vi "cXB_trt-3-sta.vi"(2 "errout":errorcluster caption="err in", 3 "cX":T1) -> (0 "err out":errorcluster, 1 "cX-s":T1)   [LabVIEW 2010]
uses:
  lv_04/commandes/cX.ctl
  lv_04/commandes/cSTA_varid.ctl
  lv_04/commandes/c_TDMS_ch_variable.ctl
  lv_04/commandes/c_TDMS_ch_donnees.ctl
  lv_04/commandes/c0-var-n.ctl
  lv_04/commandes/cSTA_num_do_cr.ctl
  lv_04/commandes/c02-do-num.ctl
  lv_04/commandes/c04-stat-num.ctl
  lv_04/commandes/cSTA_txt_do_cr.ctl
  lv_04/commandes/c02-do-txt.ctl
  lv_04/commandes/c04-stat-txt.ctl
  lv_04/commandes/cSTA_dist.ctl
  lv_04/commandes/c03-dist-S.ctl
  lv_04/commandes/c0-dist-xy.ctl
  lv_04/commandes/c03-dist-T.ctl
  lv_04/commandes/c03-dist-SPC.ctl
  lv_04/lv_04.lvlib
  lv_01/lv_01.lvlib
  lv_02/lv_02.lvlib
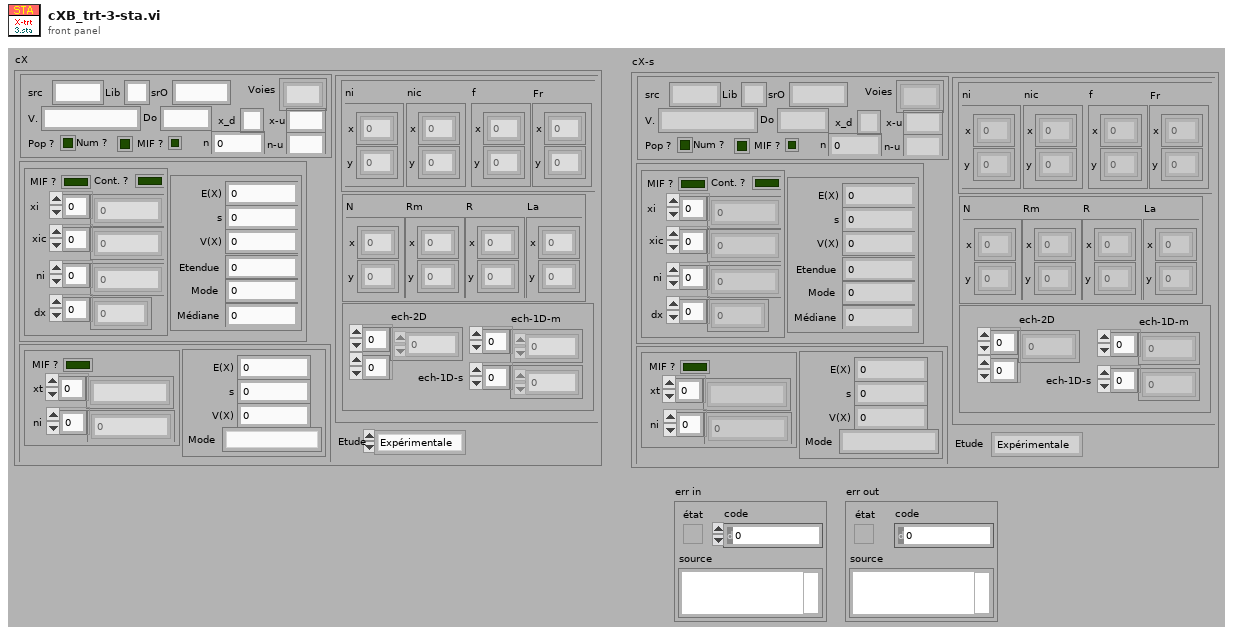
[diagram p1: front panel]
types:
  T1 = typedef "lv_04.lvlib/cX.ctl" = cluster{"src":T2, "num":T6, "txt":T9, "dist":T12, "Etude":enum16{"Expérimentale", "Modèle"}}
  T2 = typedef "lv_04.lvlib/cSTA_varid.ctl" = cluster{"src":string, "Lib":string, "srO":string, "V.":T3, "Voies":string[], "Do":T4, "n":T5, "Num ?":bool, "Pop ?":bool, "x_d":string, "x-u":string, "n-u":string, "MIF ?":bool}
  T3 = typedef "lv_04.lvlib/c_TDMS_ch_variable.ctl" = string
  T4 = typedef "lv_04.lvlib/c_TDMS_ch_donnees.ctl" = string
  T5 = typedef "lv_04.lvlib/c0-var-n.ctl" = i32
  T6 = typedef "lv_04.lvlib/cSTA_num_do_cr.ctl" = cluster{"do":T7, "sta":T8}
  T7 = typedef "lv_04.lvlib/c02-do-num.ctl" = cluster{"MIF ?":bool, "Cont. ?":bool, "xi":dbl[], "xic":dbl[], "ni":u32[], "dx":dbl[]}
  T8 = typedef "lv_04.lvlib/c04-stat-num.ctl" = cluster{"E(X)":dbl, "s":dbl, "V(X) ":dbl, "Etendue":dbl, "Mode":dbl, "Médiane":dbl}
  T9 = typedef "lv_04.lvlib/cSTA_txt_do_cr.ctl" = cluster{"do":T10, "sta":T11}
  T10 = typedef "lv_04.lvlib/c02-do-txt.ctl" = cluster{"xt":string[], "ni":dbl[], "MIF ?":bool}
  T11 = typedef "lv_04.lvlib/c04-stat-txt.ctl" = cluster{"E(X)":dbl, "s":dbl, "V(X) ":dbl, "Mode":string}
  T12 = typedef "lv_04.lvlib/cSTA_dist.ctl" = cluster{"S":T13, "T":T15, "spc":T16}
  T13 = typedef "lv_04.lvlib/c03-dist-S.ctl" = cluster{"nic":T14, "f":T14, "Fr":T14, "ni":T14}
  T14 = typedef "lv_04.lvlib/c0-dist-xy.ctl" = cluster{"x":dbl[], "y":dbl[]}
  T15 = typedef "lv_04.lvlib/c03-dist-T.ctl" = cluster{"N":T14, "Rm":T14, "R":T14, "La":T14}
  T16 = typedef "lv_04.lvlib/c03-dist-SPC.ctl" = cluster{"ech-2D":dbl[][], "ech-1D-m":dbl[], "ech-1D-s":dbl[]}
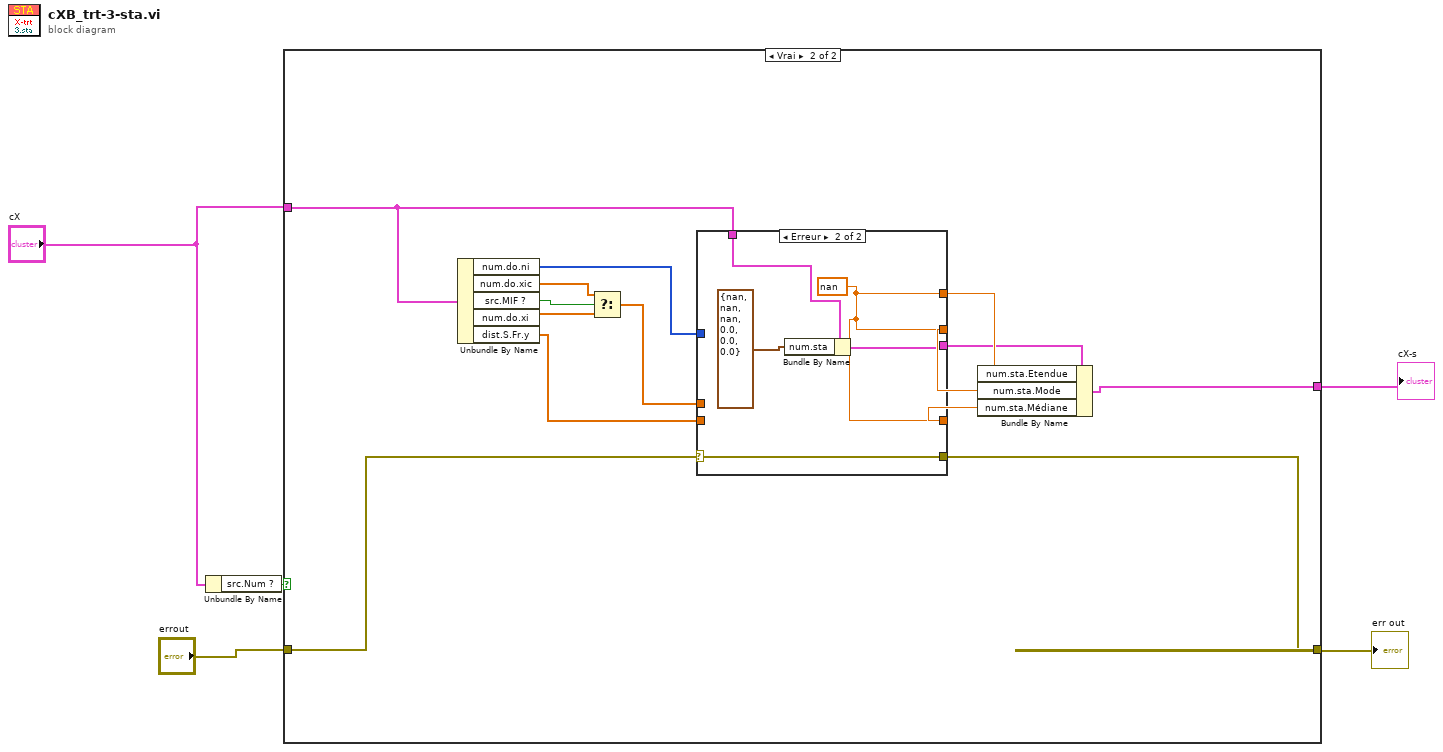
[diagram p0: block diagram]
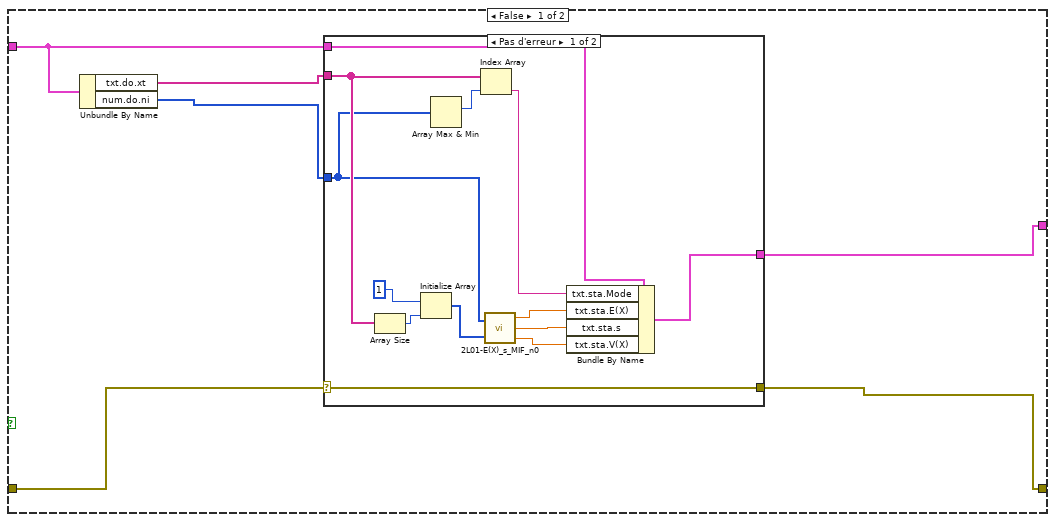
[diagram p2: hidden frame]
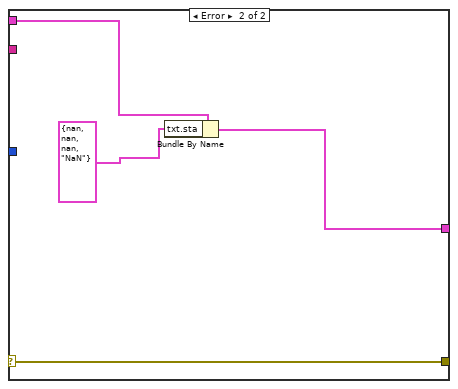
[diagram p3: hidden frame]
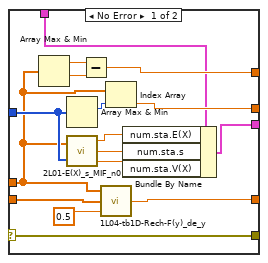
[diagram p4: hidden frame]
diagram:
  n1 = Unbundle By Name("cX") -> ("src.Num ?"=w3:bool)
  n2 = case shown="Vrai" w3 {
    tunnel: "errout" -> [w8 w30]
    tunnel: [w7 w29] -> w4
    tunnel: "cX" -> [w9 w32]
    tunnel: [w6 w33] -> w1
    frame False {
      n3 = Unbundle By Name(w9) -> ("txt.do.xt"=w11:string[], "num.do.ni"=w10:u32[])
      n4 = case shown="Pas d'erreur" w8 {
        selector: w8 -> [w23 w28]
        tunnel: [w12 w25] -> w6
        tunnel: [w23 w28] -> w7
        tunnel: w11 -> [w20 _]
        tunnel: w10 -> [w14 _]
        tunnel: w9 -> [w13 w27]
        frame No Error {
          n5 = Array Size(array=w20) -> (size(s)=w21:i32)
          n6 = Initialize Array(1, w21) -> (w22:i32[])
          n7 = Array Max & Min(array=w14) -> (max index (indices)=w24:i32)  [unwired: 3 out]
          n8 = Index Array(array=w20, index=w24) -> (element=w16:string)
          n9 = call "2L01-E(X)_s_MIF_n0.vi"("ni"=w22, "xic"=w14) -> ("V(X)"=w17:dbl, "s"=w18:dbl, "E(X)"=w19:dbl)
          n10 = Bundle By Name(cluster=w13, "txt.sta.Mode"=w16, "txt.sta.E(X)"=w19, "txt.sta.s"=w18, "txt.sta.V(X)"=w17) -> (w12:T1)
        }
        frame Error {
          n11 = Bundle By Name(cluster=w27, "txt.sta"=T11 {"E(X)"=nan, "s"=nan, "V(X) "=nan, "Mode"="NaN"} ("Car. V-TXT")) -> (w25:T1)
        }
      }
    }
    frame True {
      n12 = Unbundle By Name(w32) -> ("num.do.ni"=w42:u32[], "num.do.xic"=w38:dbl[], "src.MIF ?"=w36:bool, "num.do.xi"=w35:dbl[], "dist.S.Fr.y"=w31:dbl[])
      n13 = Select(t=w38, s=w36, f=w35) -> (s? t:f=w37:dbl[])
      n14 = case shown="Erreur" w30 {
        selector: w30 -> [w53 w63]
        tunnel: w42 -> [w52 _]
        tunnel: w37 -> [w46 _]
        tunnel: [w47 w59] -> w34
        tunnel: [w56 w62] -> w41
        tunnel: w31 -> [w45 _]
        tunnel: [w43 w62] -> w40
        tunnel: [w54 w62] -> w39
        tunnel: [w53 w63] -> w29
        tunnel: w32 -> [w48 w61]
        frame No Error {
          n15 = Array Max & Min(array=w46) -> (max value=w58:dbl, min value=w57:dbl)  [unwired: 2 out]
          n16 = Array Max & Min(array=w52) -> (max index (indices)=w55:i32)  [unwired: 3 out]
          n17 = call "2L01-E(X)_s_MIF_n0.vi"("ni"=w52, "xic"=w46) -> ("V(X)"=w49:dbl, "s"=w50:dbl, "E(X)"=w51:dbl)
          n18 = Subtract(x=w58, y=w57) -> (x-y=w56:dbl)
          n19 = call "1L04-tb1D-Rech-F(y)_de_y.vi"("y"=0.5 ("seuil y"), "F(x)"=w45, "x"=w46) -> ("F(y) interpolé"=w43:dbl)
          n20 = Index Array(array=w46, index=w55) -> (element=w54:dbl)
          n21 = Bundle By Name(cluster=w48, "num.sta.E(X)"=w51, "num.sta.s"=w50, "num.sta.V(X)"=w49) -> (w47:T1)
        }
        frame Error {
          w62 = nan
          n22 = Bundle By Name(cluster=w61, "num.sta"=T8 {"E(X)"=nan, "s"=nan, "V(X) "=nan, "Etendue"=0.0, "Mode"=0.0, "Médiane"=0.0} ("Stat. V")) -> (w59:T1)
        }
      }
      n23 = Bundle By Name(cluster=w34, "num.sta.Etendue"=w41, "num.sta.Mode"=w39, "num.sta.Médiane"=w40) -> (w33:T1)
    }
  }
  "err out" <- w4
  "cX-s" <- w1
